vi "MTecSim_Init.vi"(0 "object in":refnum<class "MTecSim.lvclass">, 5 "error in (no error)":errorcluster) -> (14 "object out":refnum<class "MTecSim.lvclass">, 19 "error out":errorcluster)   [LabVIEW 2019, in "MTecSim.lvclass"]
uses:
  MTecSim.lvclass
  MTecSim.lvclass/MTecSim.ctl
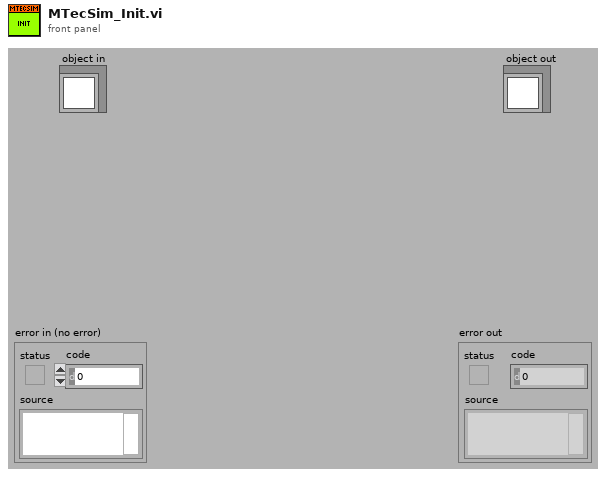
[diagram p1: front panel]
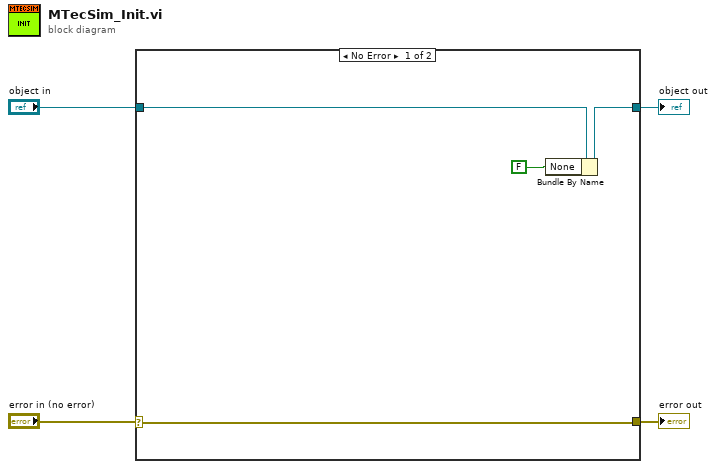
[diagram p0: block diagram]
diagram:
  n1 = case shown="No Error" "error in (no error)" {
    selector: "error in (no error)" -> [w6 w9]
    tunnel: [w8 w10] -> w4
    tunnel: "object in" -> [w5 w10]
    tunnel: [w6 w9] -> w1
    frame No Error {
      n2 = Bundle By Name(cluster=w5, "None"=FALSE) -> (w8:refnum<class "MTecSim.lvclass">)
    }
    frame Error {
    }
  }
  "object out" <- w4
  "error out" <- w1
